vi "Main.vi"(11 "Module Admin":refnum<class "Delacor_lib_QMH_Module Admin.lvclass">) -> ()   [LabVIEW 2019, in "Logging.lvlib"]
doc: "This template is based off of the Queued Message Handler design pattern and the Queued Message Handler project template that ships with LabVIEW.\n\nThe main difference is that the queue is private to this module and communication between modules is performed via Broadcast and Request events.\n\nRequest events are wrapped in public API methods and are handled in the Event Handling Loop (EHL) of this VI. Any module can register for Broadcast events sent by this module. The EHL generates messages based on user interface actions.\n\nThe Message Handling Loop (MHL) processes messages generated by the EHL, or by other messages. The messages are string values, so new messages can be added easily to the Message Cases case structure in the MHL. Each message cluster can also provide an optional value for Message Data, which is a variant that can be converted to whatever message-specific data is required.\n_____\nBased on Delacor QMH Project Template 5.0.0.82."
uses:
  Logging.lvlib
  <vilib>/Delacor/Delacor QMH/Libraries/Module Admin_class/Delacor_lib_QMH_Module Admin.lvclass
  Module Data--cluster.ctl
  <vilib>/Delacor/Delacor QMH/Libraries/Message Queue_class/Delacor_lib_QMH_Message Queue.lvclass/Delacor_lib_QMH_Message Queue.ctl
  Stop Argument--cluster.ctl
  <vilib>/Delacor/Delacor QMH/Libraries/Module Admin_class/Delacor_lib_QMH_Module Admin.lvclass/Delacor_lib_QMH_Module Admin.ctl
  Log Data Argument--cluster.ctl
  FileName Argument--cluster.ctl
  <vilib>/Utility/miscctls.llb/LVPointTypeDef.ctl
  <vilib>/Utility/sysdir.llb/System Directory Type.ctl
  <vilib>/Delacor/Delacor QMH/Libraries/Message Queue_class/Delacor_lib_QMH_Enqueue Message (Single).vi
  <vilib>/Delacor/Delacor QMH/Libraries/Module Admin_class/Delacor_lib_QMH_Get External Launch.vi
  <vilib>/Utility/error.llb/Error Cluster From Error Code.vi
  <vilib>/ErrorRing/Error Ring.xnode
  <vilib>/Delacor/Delacor QMH/Libraries/Message Queue_class/Delacor_lib_QMH_Message Queue.lvclass
panel:
  in  "Simulate MHL Error":bool
  in  "Simulate EHL Error":bool
  out "error out":errorcluster
  out "Status":string
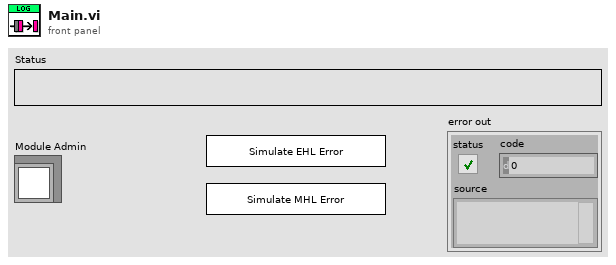
[diagram p1: front panel]
types:
  T1 = typedef "Logging.lvlib/Request Events--cluster.ctl" = cluster{"Stop Module":refnum<user-event>, "Show Panel":refnum<user-event>, "Hide Panel":refnum<user-event>, "Get Module Execution Status":refnum<user-event>, "Show Diagram":refnum<user-event>, "Log Data":refnum<user-event>, "FileName":refnum<user-event>}
  T2 = typedef "Logging.lvlib/Module Data--cluster.ctl" = cluster{"Status":string, "File Name":string}
  T3 = enum32{"invalid lock state", "Not Locked", "Locked (No Password)", "Password-protected"}
  T4 = typedef "Logging.lvlib/Stop Argument--cluster.ctl" = cluster{"Origin":string, "Exit via Stop Module Req?":bool, "Wait for Module to stop?":bool}
  T5 = typedef "Logging.lvlib/Log Data Argument--cluster.ctl" = cluster{"Log Data":string}
  T6 = typedef "Logging.lvlib/FileName Argument--cluster.ctl" = cluster{"File Name":string}
  T7 = typedef "LVPointTypeDef.ctl" = cluster{"Horizontal":i16, "Vertical":i16}
  T8 = enum32{"Invalid", "Standard", "Closed", "Hidden", "Minimized", "Maximized"}
  T9 = enum16{"open", "replace", "create", "open or create", "replace or create", "replace or create with confirmation"}
  T10 = typedef "System Directory Type.ctl" = i32
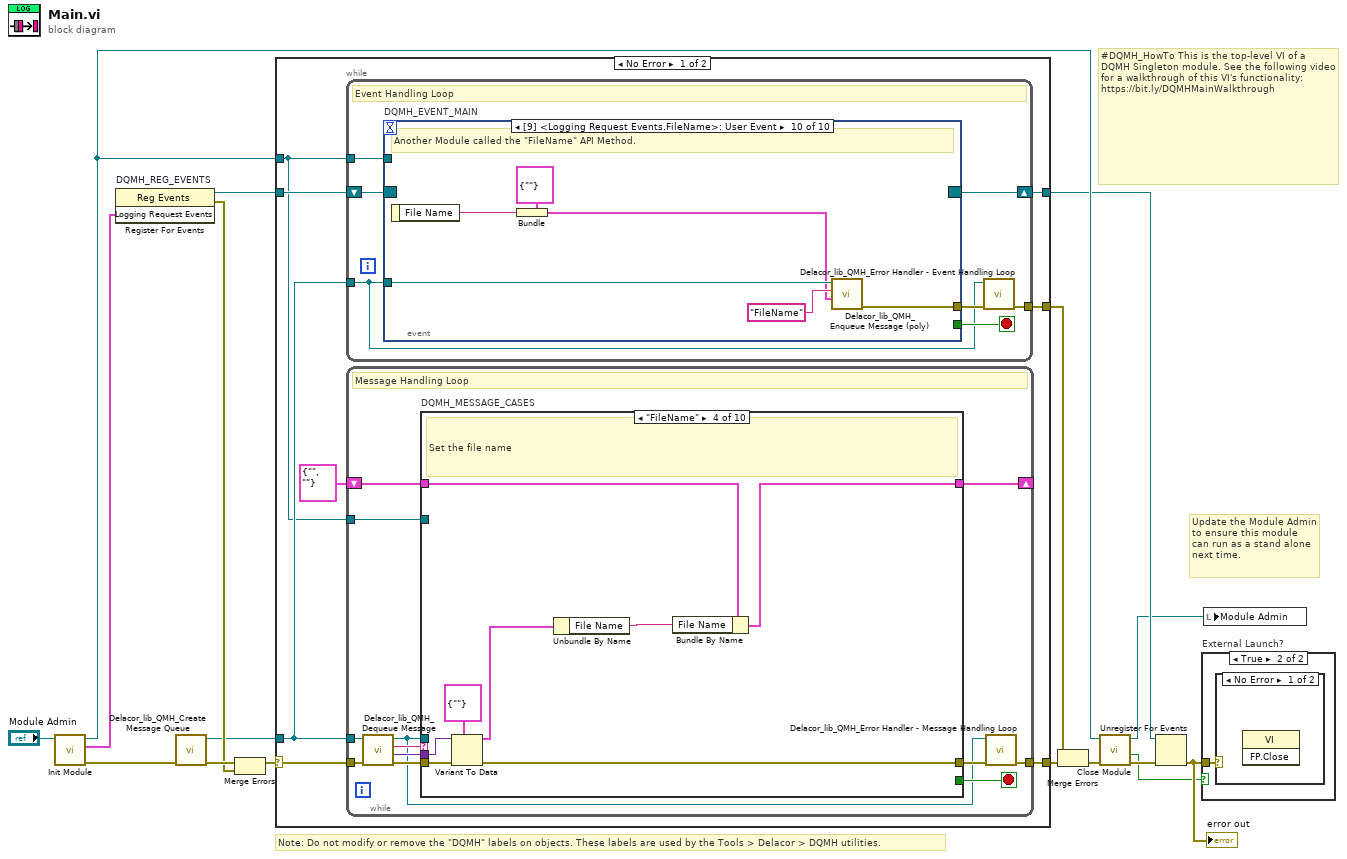
[diagram p0: block diagram]
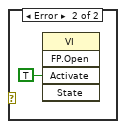
[diagram p3: hidden frame]
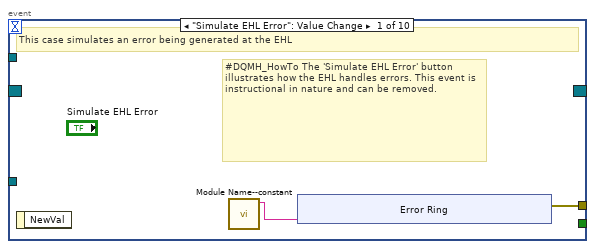
[diagram p4: hidden frame]
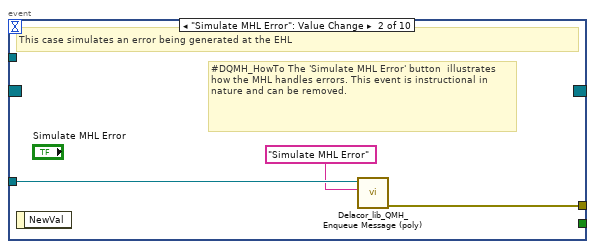
[diagram p5: hidden frame]
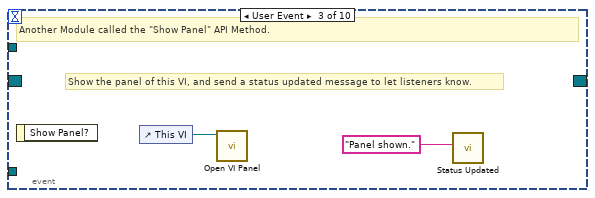
[diagram p6: hidden frame]
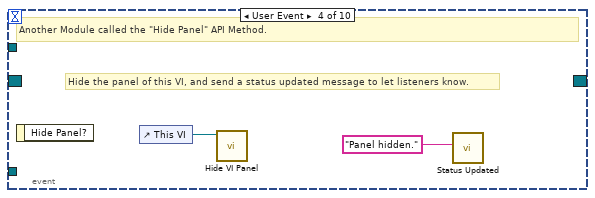
[diagram p7: hidden frame]
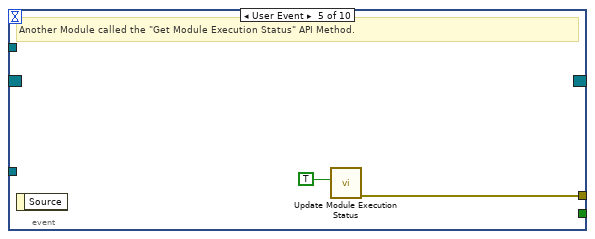
[diagram p8: hidden frame]
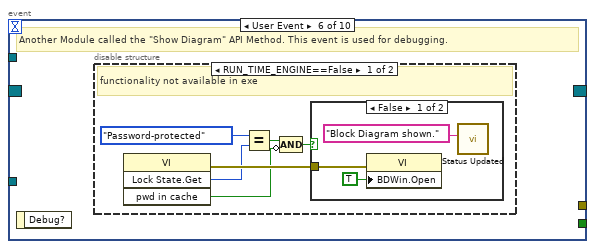
[diagram p9: hidden frame]
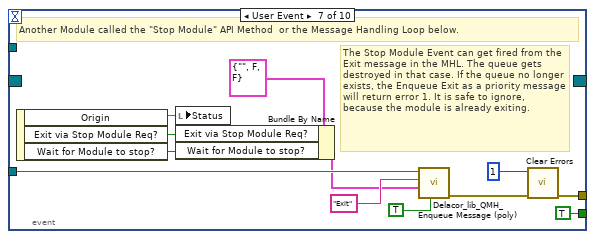
[diagram p12: hidden frame]
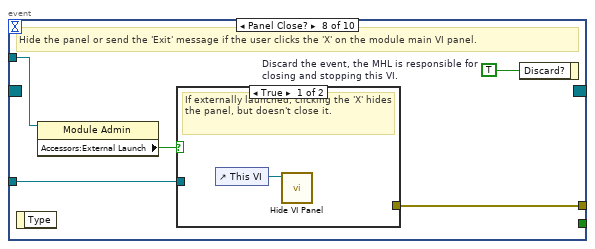
[diagram p13: hidden frame]
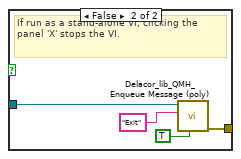
[diagram p14: hidden frame]
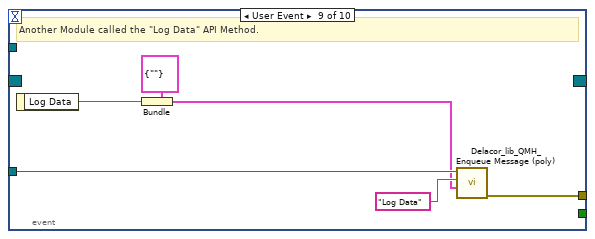
[diagram p15: hidden frame]
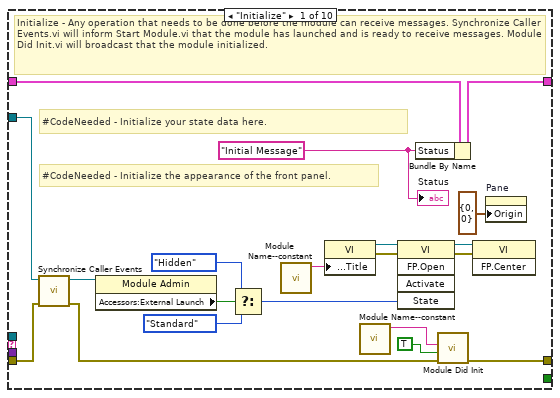
[diagram p16: hidden frame]
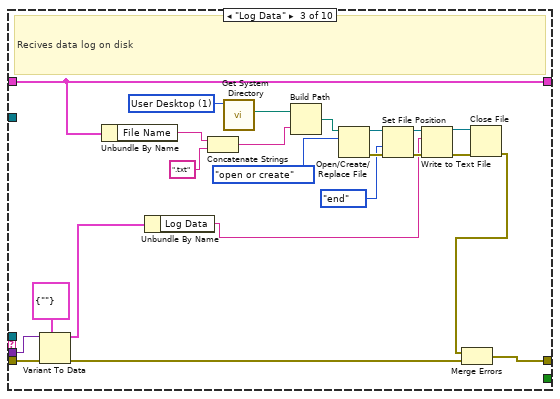
[diagram p18: hidden frame]
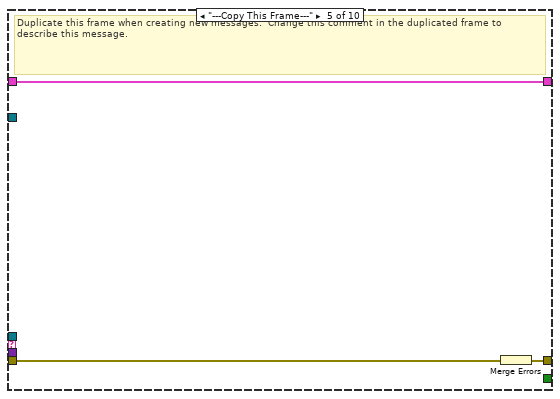
[diagram p19: hidden frame]
diagram:
  # "#DQMH_HowTo This is the top-level VI of a DQMH Singleton module. See the following video for a walkthrough of this VI's functionality: https://bit.ly/DQMHMainWalkthrough"
  # "Note: Do not modify or remove the \"DQMH\" labels on objects. These labels are used by the Tools > Delacor > DQMH utilities."
  # "Update the Module Admin to ensure this module can run as a stand alone next time."
  n1 = call "Init Module.vi"("Singleton Module Admin in"="Module Admin") -> ("error out"=w16:errorcluster, "Logging Request Events"=w5:T1, "Singleton Module Admin out"=w8:refnum<class "Delacor_lib_QMH_Module Admin.lvclass">)  [unwired: 8 in]
  n2 = register-events "DQMH_REG_EVENTS"(w5) -> (reference out=w6:refnum<event-registration>, error out=w9:errorcluster)  [unwired: 2 in]
  n3 = call <vilib>:"Delacor_lib_QMH_Create Message Queue.vi"("error in (no error)"=w16) -> ("error out"=w11:errorcluster, "Message Queue"=w4:refnum<class "Delacor_lib_QMH_Message Queue.lvclass">)  [unwired: 9 in]
  n4 = Merge Errors(w11, w9) -> (w10:errorcluster)
  n5 = case shown="No Error" w10 {
    selector: w10 -> [w23 w224]
    tunnel: [w25 w223] -> w17
    tunnel: [w22 w229] -> w7
    tunnel: w6 -> [w20 w229]
    tunnel: w4 -> [w19 w222]
    tunnel: [w24 _] -> w14
    tunnel: w8 -> [w18 w225]
    frame No Error {
      n6 = while {
        tunnel: w19 -> [w26]
        shift-right: [w29] -> w22
        shift-left: w20 -> [w30]
        tunnel: [w31] -> w24
        tunnel: w18 -> [w27]
        stop <- w28 stop-if-true
        # "Event Handling Loop"
        n7 = event "DQMH_EVENT_MAIN" shown="[9] <Logging Request Events.FileName>: User Event" {
          selector: w30 -> [_ _ _ _ _ _ _ _ _ _]
          dyn-events: [_ _ _ _ _ _ _ _ _ _] -> w29
          timeout: _ -> [_ _ _ _ _ _ _ _ _ _]
          tunnel: [_ _ _ _ _ _ TRUE ("Discard?") _ _ _] -> w28
          tunnel: w26 -> [_ w43 _ _ _ _ w67 w74 w87 w93]
          tunnel: [w34 w44 _ _ w50 _ w70 w76 w82 w88] -> w32
          tunnel: w27 -> [_ _ _ _ _ _ _ w73 _ _]
          event "Simulate EHL Error": Value Change {
            # "#DQMH_HowTo The 'Simulate EHL Error' button  illustrates how the EHL handles errors. This event is instructional in nature and can be removed."
            # "This case simulates an error being generated at the EHL"
            n8 = event-data() -> ()  [unwired: 1 in, 1 out]
            n9 = call "Module Name--constant.vi"() -> ("Module Name"=w33:string)  [unwired: 11 in]
            n10 = xnode "Error Ring"("parameter 0"=w33) -> ("error out"=w34:errorcluster)
          }
          event "Simulate MHL Error": Value Change {
            # "#DQMH_HowTo The 'Simulate MHL Error' button  illustrates how the MHL handles errors. This event is instructional in nature and can be removed."
            # "This case simulates an error being generated at the EHL"
            n11 = event-data() -> ()  [unwired: 1 in, 1 out]
            n12 = call-poly <vilib>:"Delacor_lib_QMH_Enqueue Message (poly).vi"("Message"="Simulate MHL Error", "Message Queue in"=w43) -> ("error out"=w44:errorcluster)  [unwired: 8 in, 1 out]
          }
          event User Event {
            # "Show the panel of this VI, and send a status updated message to let listeners know."
            # "Another Module called the \"Show Panel\" API Method."
            n13 = event-data() -> ()  [unwired: 1 in, 1 out]
            n14 = control-ref of="This VI"() -> (w46:refnum<vi>)
            n15 = call "Open VI Panel.vi"("VI"=w46) -> ()  [unwired: 10 in, 1 out]
            n16 = call "Status Updated.vi"("Status"="Panel shown." ("format string")) -> ()  [unwired: 10 in, 1 out]
          }
          event User Event {
            # "Hide the panel of this VI, and send a status updated message to let listeners know."
            # "Another Module called the \"Hide Panel\" API Method."
            n17 = event-data() -> ()  [unwired: 1 in, 1 out]
            n18 = control-ref of="This VI"() -> (w48:refnum<vi>)
            n19 = call "Hide VI Panel.vi"("VI"=w48) -> ()  [unwired: 10 in, 1 out]
            n20 = call "Status Updated.vi"("Status"="Panel hidden." ("format string")) -> ()  [unwired: 10 in, 1 out]
          }
          event User Event {
            # "Another Module called the \"Get Module Execution Status\" API Method."
            n21 = event-data() -> ()  [unwired: 1 in, 1 out]
            n22 = call "Update Module Execution Status.vi"("Running?"=TRUE) -> ("error out"=w50:errorcluster)  [unwired: 10 in]
          }
          event User Event {
            # "Another Module called the \"Show Diagram\" API Method. This event is used for debugging."
            n23 = event-data() -> ()  [unwired: 1 in, 1 out]
            n24 = disable-structure shown="RUN_TIME_ENGINE==False" {
              frame condition #0 (active) {
                # "functionality not available in exe"
                n25 = invoke class="VI" method="Lock State.Get"() -> (error out=w56:errorcluster, "Get Lock State"=w55:T3, "pwd in cache"=w52:bool)  [unwired: 4 in, 1 out]
                n26 = Equal?(x=T3."Password-protected", y=w55) -> (x = y?=w53:bool)
                n27 = Compound Arithmetic op=AND(w53, invert w52) -> (w51:bool)
                n28 = case shown="False" w51 {
                  tunnel: w56 -> [w59 _]
                  frame False {
                    n29 = property class="VI"(error in=w59, "BDWin.Open"=TRUE ("Block Diagram Window:Open")) -> ()  [unwired: 1 in, 2 out]
                    n30 = call "Status Updated.vi"("Status"="Block Diagram shown." ("format string")) -> ()  [unwired: 10 in, 1 out]
                  }
                  frame True {
                    # "Password-protected VI, and the password is not in the cache. Do not show the diagram."
                  }
                }
              }
              frame condition #1 {
              }
            }
          }
          event User Event {
            # "The Stop Module Event can get fired from the Exit message in the MHL. The queue gets destroyed in that case. If the queue no longer exists, the Enqueue Exit as a priority message will return error 1. It is safe to ignore, because the module is already exiting."
            # "Another Module called the \"Stop Module\" API Method  or the Message Handling Loop below."
            n31 = event-data() -> ("Origin"=w66:string, "Exit via Stop Module Req?"=w62:bool, "Wait for Module to stop?"=w61:bool)  [unwired: 1 in]
            n32 = local write "Status"(w66) -> ()
            n33 = Bundle By Name(cluster=T4 {"Origin"="", "Exit via Stop Module Req?"=FALSE, "Wait for Module to stop?"=FALSE} ("Stop Argument"), "Exit via Stop Module Req?"=w62, "Wait for Module to stop?"=w61) -> (w60:T4)
            n34 = call-poly <vilib>:"Delacor_lib_QMH_Enqueue Message (poly).vi"("Priority Message? (F)"=TRUE, "Message Data"=w60, "Message"="Exit", "Message Queue in"=w67) -> ("error out"=w71:errorcluster)  [unwired: 6 in, 1 out]
            n35 = call <vilib>:"Clear Errors.vi"("error in (no error)"=w71, "specific error code to clear (0: all)"=1) -> ("error out"=w70:errorcluster)  [unwired: 4 in, 1 out]
          }
          event Panel Close? {
            w75 = TRUE  # Discard the event, the MHL is responsible for closing and stopping this VI.
            # "Hide the panel or send the 'Exit' message if the user clicks the 'X' on the module main VI panel."
            n36 = event-data() -> ()  [unwired: 1 in, 1 out]
            n37 = property class="Module Admin"(reference=w73) -> ("Accessors:External Launch"=w72:bool)  [unwired: 1 in, 2 out]
            n38 = case shown="True" w72 {
              tunnel: w74 -> [_ w80]
              tunnel: [_ w81] -> w76
              frame True {
                # "If externally launched, clicking the 'X' hides the panel, but doesn't close it."
                n39 = control-ref of="This VI"() -> (w77:refnum<vi>)
                n40 = call "Hide VI Panel.vi"("VI"=w77) -> ()  [unwired: 10 in, 1 out]
              }
              frame False {
                # "If run as a stand-alone VI, clicking the panel 'X' stops the VI."
                n41 = call-poly <vilib>:"Delacor_lib_QMH_Enqueue Message (poly).vi"("Priority Message? (F)"=TRUE, "Message"="Exit", "Message Queue in"=w80) -> ("error out"=w81:errorcluster)  [unwired: 7 in, 1 out]
              }
            }
            n42 = event-data("Discard?"=w75) -> ()  [unwired: 1 in, 1 out]
          }
          event User Event {
            # "Another Module called the \"Log Data\" API Method."
            n43 = event-data() -> ("Log Data"=w83:string)  [unwired: 1 in]
            n44 = Bundle(cluster=T5 {"Log Data"=""} ("Log Data Argument"), "Log Data"=w83) -> (w84:T5)
            n45 = call-poly <vilib>:"Delacor_lib_QMH_Enqueue Message (poly).vi"("Message Data"=w84, "Message"="Log Data", "Message Queue in"=w87) -> ("error out"=w82:errorcluster)  [unwired: 7 in, 1 out]
          }
          event User Event {
            # "Another Module called the \"FileName\" API Method."
            n46 = event-data() -> ("File Name"=w89:string)  [unwired: 1 in]
            n47 = Bundle(cluster=T6 {"File Name"=""} ("FileName Argument"), "File Name"=w89) -> (w90:T6)
            n48 = call-poly <vilib>:"Delacor_lib_QMH_Enqueue Message (poly).vi"("Message Data"=w90, "Message"="FileName", "Message Queue in"=w93) -> ("error out"=w88:errorcluster)  [unwired: 7 in, 1 out]
          }
        }
        n49 = call-dynamic "Delacor_lib_QMH_Error Handler - Event Handling Loop.vi"("error in (no error)"=w32, "Message Queue in"=w26) -> ("dup error in"=w31:errorcluster)  [unwired: 8 in, 1 out]
      }
      n50 = while {
        tunnel: w19 -> [w96]
        shift-right: [w100] -> _
        shift-left: T2 {"Status"="", "File Name"=""} ("Data Cluster") -> [w101]
        tunnel: w23 -> [w104]
        tunnel: [w102] -> w25
        tunnel: w18 -> [w94]
        stop <- w99 stop-if-true
        # "Message Handling Loop"
        n51 = call-dynamic "Delacor_lib_QMH_Dequeue Message.vi"("error in (no error)"=w104, "Message Queue in"=w96) -> ("error out"=w103:errorcluster, "Message Data"=w97:variant, "Message"=w98:string, "Message Queue out"=w95:refnum<class "Delacor_lib_QMH_Message Queue.lvclass">)  [unwired: 6 in]
        n52 = case "DQMH_MESSAGE_CASES" shown="\"FileName\"" w98 {
          selector: w98 -> [_ _ _ _ _ _ _ _ _ w209]
          tunnel: w95 -> [_ _ _ _ _ _ _ w179 w201 _]
          tunnel: w103 -> [w123 w127 w150 w158 w161 w163 w168 w186 w207 w211]
          tunnel: [w121 w127 w130 w157 w160 w163 w167 w182 w204 w212] -> w105
          tunnel: w101 -> [w112 w126 w146 w153 w159 w162 w165 w181 w200 w210]
          tunnel: [w111 w126 w146 w152 w159 w162 w165 w181 w200 w210] -> w100
          tunnel: [_ _ _ _ _ _ _ _ w199 _] -> w99
          tunnel: w97 -> [_ _ w149 w156 _ _ _ w180 w198 _]
          tunnel: w94 -> [w113 _ _ _ _ _ _ w178 w193 _]
          frame "Initialize" {
            w106 = "Initial Message" ("Initial Message")
            # "#CodeNeeded - Initialize the appearance of the front panel."
            # "#CodeNeeded - Initialize your state data here."
            # "Initialize - Any operation that needs to be done before the module can receive messages. Synchronize Caller Events.vi will inform Start Module.vi that the module has launched and is ready to receive messages. Module Did Init.vi will broadcast that the module initialized."
            n53 = call "Synchronize Caller Events.vi"("error in (no error)"=w123, "Singleton Module Admin in"=w113) -> ("error out"=w122:errorcluster, "Singleton Module Admin out"=w108:refnum<class "Delacor_lib_QMH_Module Admin.lvclass">)  [unwired: 8 in]
            n54 = property class="Module Admin"(reference=w108) -> ("Accessors:External Launch"=w117:bool)  [unwired: 1 in, 2 out]
            n55 = Select(t=T8."Hidden" ("State"), s=w117, f=T8."Standard" ("State")) -> (s? t:f=w114:T8)
            n56 = call "Module Name--constant.vi"() -> ("Module Name"=w120:string)  [unwired: 11 in]
            n57 = property class="VI"("Front Panel.Title"=w120) -> (reference out=w119:refnum<vi>, error out=w125:errorcluster)  [unwired: 2 in]
            n58 = call "Module Name--constant.vi"() -> ("Module Name"=w109:string)  [unwired: 11 in]
            n59 = invoke class="VI" method="FP.Open"(reference=w119, error in=w125, "State"=w114) -> (reference out=w118:refnum<vi>, error out=w124:errorcluster)  [unwired: 2 in, 3 out]
            n60 = Bundle By Name(cluster=w112, "Status"=w106) -> (w111:T2)
            n61 = call "Module Did Init.vi"("error in (no error)"=w122, "Initialized?"=TRUE, "Origin"=w109) -> ("error out"=w121:errorcluster)  [unwired: 8 in]
            n62 = invoke class="VI" method="FP.Center"(reference=w118, error in=w124) -> ()  [unwired: 1 in, 3 out]
            n63 = property on="Pane" class="Pane"("Origin"=T7 {"Horizontal"=0, "Vertical"=0}) -> ()  [unwired: 2 in, 2 out]
            "Status" <- w106
          }
          frame "--- Module Specific ---" {
            # "Separator -- The following cases handle messages specific to this Module."
          }
          frame "Log Data" {
            w145 = T10 1 items=["User Home"=0, "User Desktop"=1, "User Documents"=2, "User Application Data"=3, "User Preferences"=4, "User Temporary"=5, "Public Documents"=6, "Public Application Data"=7, "Public Preferences"=8, "Public Cache"=13, "System Core Libraries"=9, "System Installed Libraries"=10, "Application Files"=11, "Boot Volume Root"=12] ("system directory type")
            # "Recives data log on disk"
            n64 = Variant To Data(error in=w150, type=T5 {"Log Data"=""} ("Log Data Argument"), Variant=w149) -> (data=w147:T5, error out=w129:errorcluster)
            n65 = Unbundle By Name(w146) -> ("File Name"=w142:string)
            n66 = Unbundle By Name(w147) -> ("Log Data"=w131:string)
            n67 = Concatenate Strings(w142, ".txt" ("string")) -> (w143:string)
            n68 = call <vilib>:"Get System Directory.vi"("system directory type"=w145) -> ("system directory"=w144:path)  [unwired: 10 in]
            n69 = Build Path(base path=w144, name or relative path=w143) -> (appended path=w140:path)
            n70 = Open/Create/Replace File(file path (use dialog)=w140, operation (0:open)=T9."open or create") -> (refnum out=w133:refnum<file>, error out=w138:errorcluster)  [unwired: 4 in, 1 out]
            n71 = Set File Position(refnum=w133, from (0:start)=enum16{"start", "end", "current"}."end", error in=w138) -> (refnum out=w134:refnum<file>, error out=w137:errorcluster)  [unwired: 1 in]
            n72 = Write to Text File(file (use dialog)=w134, text=w131, error in=w137) -> (refnum out=w135:refnum<file>, error out=w136:errorcluster)  [unwired: 1 in, 1 out]
            n73 = Close File(refnum=w135, error in=w136) -> (error out=w128:errorcluster)  [unwired: 1 out]
            n74 = Merge Errors(w128, w129) -> (w130:errorcluster)
          }
          frame "FileName" {
            # "Set the file name"
            n75 = Variant To Data(error in=w158, type=T6 {"File Name"=""} ("FileName Argument"), Variant=w156) -> (data=w154:T6, error out=w157:errorcluster)
            n76 = Unbundle By Name(w154) -> ("File Name"=w151:string)
            n77 = Bundle By Name(cluster=w153, "File Name"=w151) -> (w152:T2)
          }
          frame "---Copy This Frame---" {
            # "Duplicate this frame when creating new messages.  Change this comment in the duplicated frame to describe this message."
            n78 = Merge Errors(w161) -> (w160:errorcluster)
          }
          frame "--- Exit and Error Handling---" {
            # "Separator - The following cases handle errors and exit messages."
          }
          frame "Simulate MHL Error" {
            # "#DQMH_HowTo The 'Simulate MHL Error' button  illustrates how the MHL handles errors. This event is instructional in nature and can be removed."
            # "Simulate an error occurring at the MHL"
            n79 = call "Module Name--constant.vi"() -> ("Module Name"=w164:string)  [unwired: 11 in]
            n80 = xnode "Error Ring"("parameter 0"=w164) -> ("error out"=w166:errorcluster)
            n81 = Merge Errors(w168, w166) -> (w167:errorcluster)
          }
          frame "Error" {
            # "#CodeRecommended - If you ever change the name of this \"Error\" message, you'll need to update the name in the Check Loop Error.vi as well."
            # "#CodeRecommended - If the module is running in standalone mode (External Launch = FALSE), this code will pop up an error dialog and call the 'Exit' message if an error occurs. Add more fine-grained error handling here."
            # "Error - Check the error message data and respond accordingly. This message is sent by the \"Error Handler\" VIs at the end of each loop in this application."
            n82 = property class="Module Admin"(reference=w178) -> ("Accessors:External Launch"=w177:bool)  [unwired: 1 in, 2 out]
            n83 = Variant To Data(error in=w186, type=errorcluster {"status"=FALSE, "code"=0, "source"=""} ("error constant"), Variant=w180) -> (data=w187:errorcluster, error out=w184:errorcluster)
            n84 = call "Module Name--constant.vi"() -> ("Module Name"=w176:string)  [unwired: 11 in]
            n85 = call "Error Reported.vi"("Additional Information"=w176, "Error"=w187) -> ()  [unwired: 9 in, 1 out]
            n86 = case shown="False" w177 {
              tunnel: [w192 _] -> w183
              tunnel: w179 -> [w190 _]
              tunnel: w187 -> [w191 _]
              frame False {
                # "If the module is running standalone, then pop up an error dialog and call the \"Exit\" message."
                n87 = call <vilib>:"Simple Error Handler.vi"("error in (no error)"=w191) -> ()  [unwired: 4 in, 5 out]
                n88 = call-poly <vilib>:"Delacor_lib_QMH_Enqueue Message (poly).vi"("Priority Message? (F)"=TRUE, "Message"="Exit", "Message Queue in"=w190) -> ("error out"=w192:errorcluster)  [unwired: 7 in, 1 out]
              }
              frame True {
                # "If the module was launched externally, calling the Error Reported broadcast VI is the only action performed by the \"Error\" message. The module's caller can then process the error appropriately."
              }
            }
            n89 = Merge Errors(w184, w183) -> (w182:errorcluster)
            n90 = local write "error out"(w182) -> ()
          }
          frame "Exit" {
            w197 = 91  # 91: not all Exit messages will have an argument
            w199 = TRUE  # Stop the VI
            # "Release the message queue reference"
            # "#CodeNeeded - Add any required cleanup code here"
            # "Exit - Exit the application."
            n91 = Variant To Data(error in=w207, type=T4 {"Origin"="", "Exit via Stop Module Req?"=FALSE, "Wait for Module to stop?"=FALSE} ("Stop Argument"), Variant=w198) -> (data=w195:T4, error out=w203:errorcluster)
            n92 = call <vilib>:"Clear Errors.vi"("error in (no error)"=w203, "specific error code to clear (0: all)"=w197) -> ("error out"=w206:errorcluster)  [unwired: 4 in, 1 out]
            n93 = control-ref of="This VI"() -> (w194:refnum<vi>)
            n94 = call-dynamic "Delacor_lib_QMH_Release Message Queue.vi"("error in (no error)"=w206, "Message Queue"=w201) -> ("error out"=w205:errorcluster)  [unwired: 9 in]
            n95 = call "Handle Exit.vi"("Stop Argument"=w195, "Admin in"=w193, "VI reference"=w194) -> ("error out"=w202:errorcluster)  [unwired: 7 in, 1 out]
            n96 = Merge Errors(w205, w202) -> (w204:errorcluster)
          }
          frame Default {
            # "'Default' case only runs if there is a message that isn't defined in any of the other cases.  Output a programming error."
            n97 = call "Module Name--constant.vi"() -> ("Module Name"=w208:string)  [unwired: 11 in]
            n98 = xnode "Error Ring"("parameter 0"=w209, "parameter 1"=w208) -> ("error out"=w213:errorcluster)
            n99 = Merge Errors(w211, w213) -> (w212:errorcluster)
          }
        }
        n100 = call-dynamic "Delacor_lib_QMH_Error Handler - Message Handling Loop.vi"("error in (no error)"=w105, "Message Queue in"=w95) -> ("dup error in"=w102:errorcluster)  [unwired: 8 in, 1 out]
      }
    }
    frame Error {
      # "Synchronize Caller Events.vi will inform Start Module.vi that the module has launched and will let the code calling Start Module.vi register for broadcasts and would permit the caller receive the broadcast that an error occurred at launch time."
      n101 = call-dynamic "Delacor_lib_QMH_Release Message Queue.vi"("error in (no error)"=w224, "Message Queue"=w222) -> ("error out"=w223:errorcluster)  [unwired: 9 in]
      n102 = call "Synchronize Caller Events.vi"("Singleton Module Admin in"=w225) -> ("error out"=w230:errorcluster)  [unwired: 9 in, 1 out]
      n103 = call "Module Name--constant.vi"() -> ("Module Name"=w228:string)  [unwired: 11 in]
      n104 = Format Into String(format string="An error occurred during initialization. %s is no longer running.", w228) -> (resulting string=w226:string)  [unwired: 2 in, 1 out]
      n105 = Merge Errors(w223, w230) -> (w231:errorcluster)
      n106 = call "Error Reported.vi"("Additional Information"=w226, "Error"=w231) -> ()  [unwired: 9 in, 1 out]
    }
  }
  n107 = Merge Errors(w14, w17) -> (w13:errorcluster)
  n108 = call "Close Module.vi"("error in (no error)"=w13, "Module Admin in"=w8) -> ("error out"=w15:errorcluster, "External Launch"=w1:bool, "Module Admin out"=w2:refnum<class "Delacor_lib_QMH_Module Admin.lvclass">)  [unwired: 7 in]
  n109 = Unregister For Events(event registration refnum=w7, error in=w15) -> (error out=w12:errorcluster)
  "error out" <- w12
  n110 = case "External Launch?" shown="True" w1 {
    tunnel: w12 -> [_ w232]
    frame False {
    }
    frame True {
      n111 = case shown="No Error" w232 {
        frame No Error {
          n112 = invoke class="VI" method="FP.Close"() -> ()  [unwired: 3 in, 3 out]
        }
        frame Error {
          n113 = invoke class="VI" method="FP.Open"("Activate"=TRUE ("Activate?")) -> ()  [unwired: 4 in, 5 out]
        }
      }
    }
  }
  n114 = local write "Module Admin"(w2) -> ()
